vi "Close Facade.vi"(8 "error in":errorcluster, 11 "GUI Facade in":refnum<class "GUI Facade.lvclass">) -> (0 "error out":errorcluster, 3 "GUI Facade out":refnum<class "GUI Facade.lvclass">)   [LabVIEW 2018, in "GUI Facade.lvclass"]
doc: "Send the stop signal to the open UIs, close the data references, remove the current VI from the subpanel and close the reference to all of the panels."
uses:
  GUI Facade.lvclass
  GUI.lvclass
  Observer/Data Subject.lvclass
  File IO/Class/File Observer.lvclass
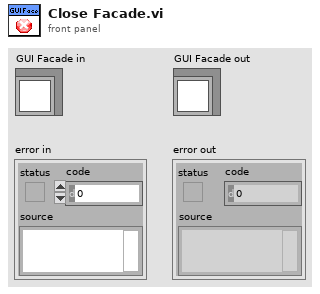
[diagram p1: front panel]
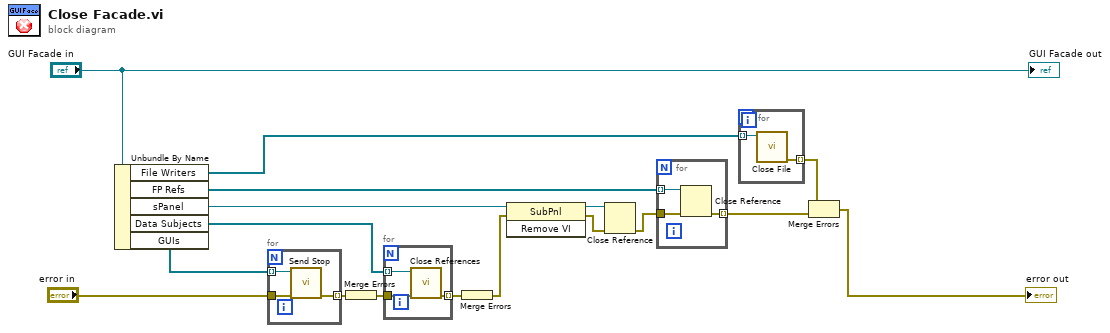
[diagram p0: block diagram]
diagram:
  n1 = Unbundle By Name("GUI Facade in") -> ("File Writers"=w2:refnum<class "File Observer.lvclass">[], "FP Refs"=w7:refnum<vi>[], "sPanel"=w13:refnum<vi>, "Data Subjects"=w10:refnum<class "Data Subject.lvclass">[], "GUIs"=w11:refnum<class "GUI.lvclass">[])
  n2 = for {
    tunnel: [w20] -> w14 mode=indexing
    tunnel: w11 -> [w19] mode=indexing
    tunnel: "error in" -> [w18]
    n3 = call "Send Stop.vi"("error in"=w18, "GUI in"=w19) -> ("error out"=w20:errorcluster)  [unwired: 8 in, 1 out]
  }
  n4 = Merge Errors(w14) -> (w12:errorcluster)
  n5 = for {
    tunnel: w12 -> [w23]
    tunnel: w10 -> [w22] mode=indexing
    tunnel: [w21] -> w9 mode=indexing
    n6 = call "Close References.vi"("error in"=w23, "Data Subject in"=w22) -> ("error out"=w21:errorcluster)  [unwired: 8 in, 1 out]
  }
  n7 = Merge Errors(w9) -> (w8:errorcluster)
  n8 = invoke class="SubPnl" method="Remove VI"(reference=w13, error in=w8) -> (reference out=w5:refnum<vi>, error out=w4:errorcluster)  [unwired: 1 in, 1 out]
  n9 = Close Reference(reference=w5, error in (no error)=w4) -> (error out=w3:errorcluster)
  n10 = for {
    tunnel: w7 -> [w26] mode=indexing
    tunnel: w3 -> [w25]
    tunnel: [w24] -> w6 mode=indexing
    n11 = Close Reference(reference=w26, error in (no error)=w25) -> (error out=w24:errorcluster)
  }
  n12 = for {
    tunnel: w2 -> [w28] mode=indexing
    tunnel: [w27] -> w1 mode=indexing
    n13 = call-dynamic "Close File.vi"("File Obs in"=w28) -> ("error out"=w27:errorcluster)  [unwired: 9 in, 1 out]
  }
  n14 = Merge Errors(w1, w6) -> (→"error out":errorcluster)
  "GUI Facade out" <- "GUI Facade in"
